vi "LoopselFFBlock.VI"() -> ()   [LabVIEW 2015]
panel:
  in  "no.of blocks":u32=2
  out "SEC":dbl=0.0202
  out "MB RAM":u32=4
  in  "?":enum32{"1", "2", "3"}(radio)=enum."3"
  in  "pos slope":u8=1
  in  "both slopes":u8
  in  "DAT in 10ns":u32
  out "FIFO overflow":bool
  in  "extTrig 0/1":u8
  in  "Start Read":bool
  in  "stop all":bool
  in  "Arm/Clear arry":bool
  in  "Slide":u32(slide)=1010 scale=996.0..1030.0
  in  "frequency[Hz]":u32
  in  "no.of samples (nos)":u32=1010
  in  "exposuretime[ms]":dbl=0.02 format="%.3f"
  out "Signalverlaufgraph":u16[](graph)=[542, 542, 543, 543, 0, 0, 1009, 0, 2, 2, 3, 3, 4, 4, 5, 5, 6, 6, 7, 7, 8, 8, 9, 9, 10, 10, 11, 11, 12, 12, 13, 13, 14, 14, 15, 15, 16, 16, 17, 17, 18, 18, 19, 19, 20, 20, 21, 21, 22, 22, 23, 23, 24, 24, 25, 25, 26, 26, 27, 27, 28, 28, 29, 29, 30, 30, 31, 31, 32, 32, 33, 33, 34, 34, 35, 35, 36, 36, 37, 37, 38, 38, 39, 39, 40, 40, 41, 41, 42, 42, 43, 43, 44, 44, 45, 45, 46, 46, 47, 47, 48, 48, 49, 49, 50, 50, 51, 51, 52, 52, 53, 53, 54, 54, 55, 55, 56, 56, 57, 57, 58, 58, 59, 59, 60, 60, 61, 61, 62, 62, 63, 63, 64, 64, 65, 65, 66, 66, 67, 67, 68, 68, 69, 69, 70, 70, 71, 71, 72, 72, 73, 73, 74, 74, 75, 75, 76, 76, 77, 77, 78, 78, 79, 79, 80, 80, 81, 81, 82, 82, 83, 83, 84, 84, 85, 85, 86, 86, 87, 87, 88, 88, 89, 89, 90, 90, 91, 91, 92, 92, 93, 93, 94, 94, 95, 95, 96, 96, 97, 97, 98, 98, 99, 99, 100, 100, 101, 101, 102, 102, 103, 103, 104, 104, 105, 105, 106, 106, 107, 107, 108, 108, 109, 109, 110, 110, 111, 111, 112, 112, 113, 113, 114, 114, 115, 115, 116, 116, 117, 117, 118, 118, 119, 119, 120, 120, 121, 121, 122, 122, 123, 123, 124, 124, 125, 125, 126, 126, 127, 127, 128, 128, 129, 129, 130, 130, 131, 131, 132, 132, 133, 133, 134, 134, 135, 135, 136, 136, 137, 137, 138, 138, 139, 139, 140, 140, 141, 141, 142, 142, 143, 143, 144, 144, 145, 145, 146, 146, 147, 147, 148, 148, 149, 149, 150, 150, 151, 151, 152, 152, 153, 153, 154, 154, 155, 155, 156, 156, 157, 157, 158, 158, 159, 159, 160, 160, 161, 161, 162, 162, 163, 163, 164, 164, 165, 165, 166, 166, 167, 167, 168, 168, 169, 169, 170, 170, 171, 171, 172, 172, 173, 173, 174, 174, 175, 175, 176, 176, 177, 177, 178, 178, 179, 179, 180, 180, 181, 181, 182, 182, 183, 183, 184, 184, 185, 185, 186, 186, 187, 187, 188, 188, 189, 189, 190, 190, 191, 191, 192, 192, 193, 193, 194, 194, 195, 195, 196, 196, 197, 197, 198, 198, 199, 199, 200, 200, 201, 201, 202, 202, 203, 203, 204, 204, 205, 205, 206, 206, 207, 207, 208, 208, 209, 209, 210, 210, 211, 211, 212, 212, 213, 213, 214, 214, 215, 215, 216, 216, 217, 217, 218, 218, 219, 219, 220, 220, 221, 221, 222, 222, 223, 223, 224, 224, 225, 225, 226, 226, 227, 227, 228, 228, 229, 229, 230, 230, 231, 231, 232, 232, 233, 233, 234, 234, 235, 235, 236, 236, 237, 237, 238, 238, 239, 239, 240, 240, 241, 241, 242, 242, 243, 243, 244, 244, 245, 245, 246, 246, 247, 247, 248, 248, 249, 249, 250, 250, 251, 251, 252, 252, 253, 253, 254, 254, 255, 255, 256, 256, 257, 257, 258, 258, 259, 259, 260, 260, 261, 261, 262, 262, 263, 263, 264, 264, 265, 265, 266, 266, 267, 267, 268, 268, 269, 269, 270, 270, 271, 271, 272, 272, 273, 273, 274, 274, 275, 275, 276, 276, 277, 277, 278, 278, 279, 279, 280, 280, 281, 281, 282, 282, 283, 283, 284, 284, 285, 285, 286, 286, 287, 287, 288, 288, 289, 289, 290, 290, 291, 291, 292, 292, 293, 293, 294, 294, 295, 295, 296, 296, 297, 297, 298, 298, 299, 299, 300, 300, 301, 301, 302, 302, 303, 303, 304, 304, 305, 305, 306, 306, 307, 307, 308, 308, 309, 309, 310, 310, 311, 311, 312, 312, 313, 313, 314, 314, 315, 315, 316, 316, 317, 317, 318, 318, 319, 319, 320, 320, 321, 321, 322, 322, 323, 323, 324, 324, 325, 325, 326, 326, 327, 327, 328, 328, 329, 329, 330, 330, 331, 331, 332, 332, 333, 333, 334, 334, 335, 335, 336, 336, 337, 337, 338, 338, 339, 339, 340, 340, 341, 341, 342, 342, 343, 343, 344, 344, 345, 345, 346, 346, 347, 347, 348, 348, 349, 349, 350, 350, 351, 351, 352, 352, 353, 353, 354, 354, 355, 355, 356, 356, 357, 357, 358, 358, 359, 359, 360, 360, 361, 361, 362, 362, 363, 363, 364, 364, 365, 365, 366, 366, 367, 367, 368, 368, 369, 369, 370, 370, 371, 371, 372, 372, 373, 373, 374, 374, 375, 375, 376, 376, 377, 377, 378, 378, 379, 379, 380, 380, 381, 381, 382, 382, 383, 383, 384, 384, 385, 385, 386, 386, 387, 387, 388, 388, 389, 389, 390, 390, 391, 391, 392, 392, 393, 393, 394, 394, 395, 395, 396, 396, 397, 397, 398, 398, 399, 399, 400, 400, 401, 401, 402, 402, 403, 403, 404, 404, 405, 405, 406, 406, 407, 407, 408, 408, 409, 409, 410, 410, 411, 411, 412, 412, 413, 413, 414, 414, 415, 415, 416, 416, 417, 417, 418, 418, 419, 419, 420, 420, 421, 421, 422, 422, 423, 423, 424, 424, 425, 425, 426, 426, 427, 427, 428, 428, 429, 429, 430, 430, 431, 431, 432, 432, 433, 433, 434, 434, 435, 435, 436, 436, 437, 437, 438, 438, 439, 439, 440, 440, 441, 441, 442, 442, 443, 443, 444, 444, 445, 445, 446, 446, 447, 447, 448, 448, 449, 449, 450, 450, 451, 451, 452, 452, 453, 453, 454, 454, 455, 455, 456, 456, 457, 457, 458, 458, 459, 459, 460, 460, 461, 461, 462, 462, 463, 463, 464, 464, 465, 465, 466, 466, 467, 467, 468, 468, 469, 469, 470, 470, 471, 471, 472, 472, 473, 473, 474, 474, 475, 475, 476, 476, 477, 477, 478, 478, 479, 479, 480, 480, 481, 481, 482, 482, 483, 483, 484, 484, 485, 485, 486, 486, 487, 487, 488, 488, 489, 489, 490, 490, 491, 491, 492, 492, 493, 493, 494, 494, 495, 495, 496, 496, 497, 497, 498, 498, 499, 499, 500, 500, 501, 501, 502, 502, 503, 503, 504, 504, 505, 505, 506, 506, 507, 507, 508, 508, 509, 509, 510, 510, 511, 511, 512, 512, 513, 513, 514, 514, 515, 515, 516, 516, 517, 517, 518, 518, 519, 519, 520, 520, 521, 521, 522, 522, 523, 523, 524, 524, 525, 525, 526, 526, 527, 527, 528, 528, 529, 529, 530, 530, 531, 531, 532, 532, 533, 533, 534, 534, 535, 535, 536, 536, 537, 537, 538, 538, 539, 539, 540, 540, 541, 541]
  # "Start with run"
  # "Abort with ESC"
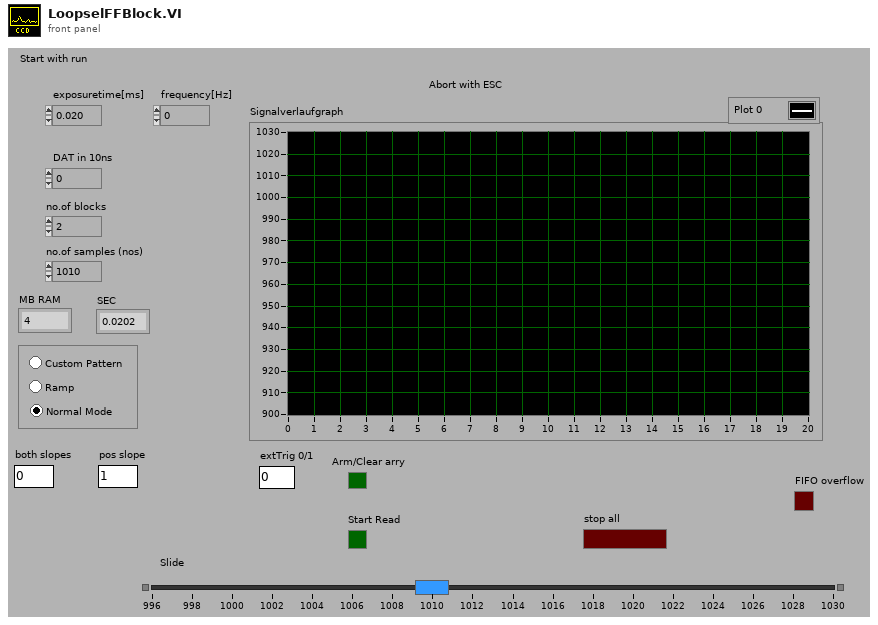
[diagram p1: front panel]
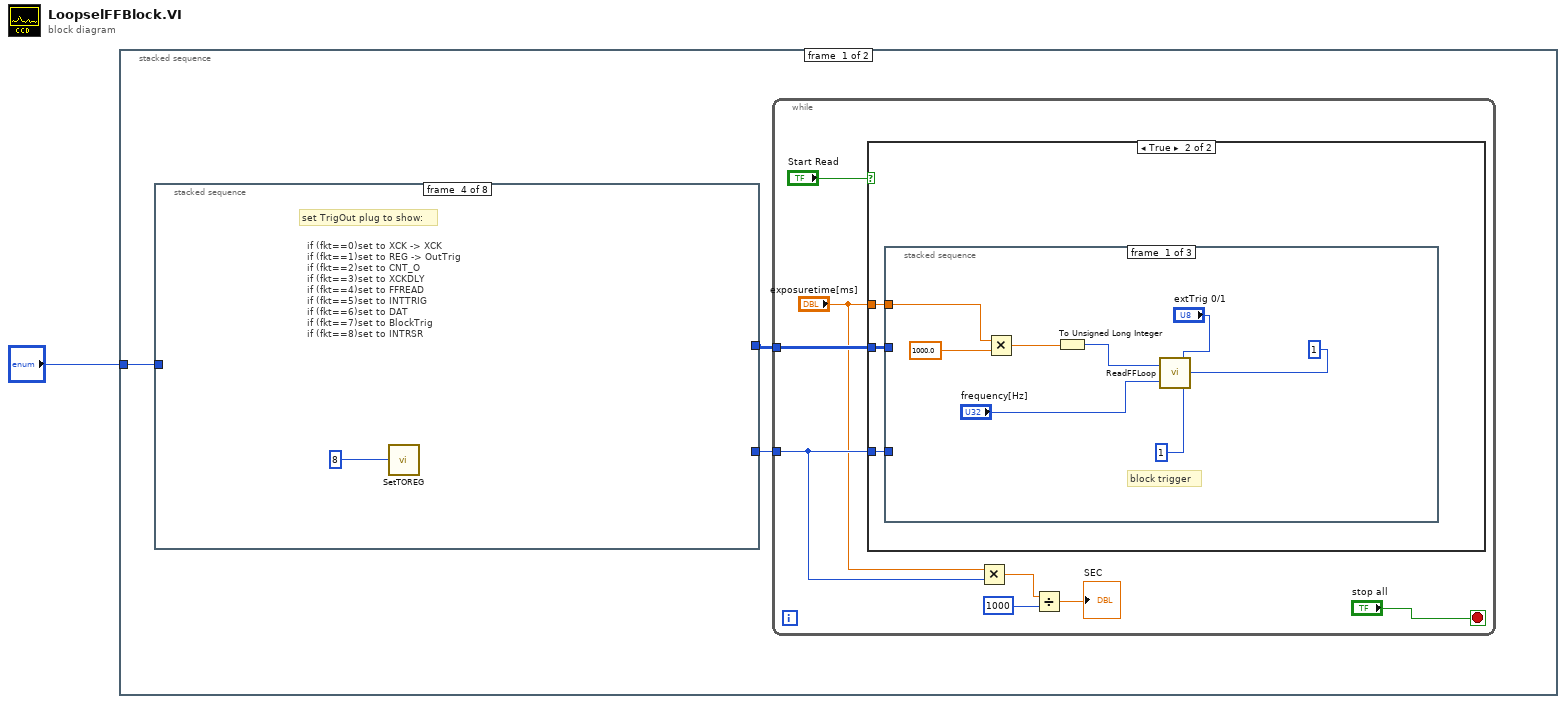
[diagram p0: block diagram]
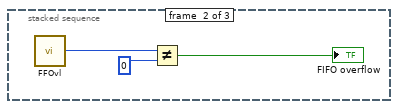
[diagram p3: hidden frame]
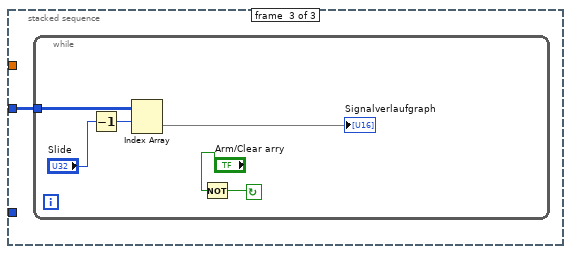
[diagram p4: hidden frame]
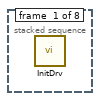
[diagram p5: hidden frame]
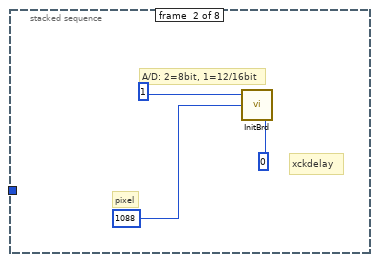
[diagram p6: hidden frame]
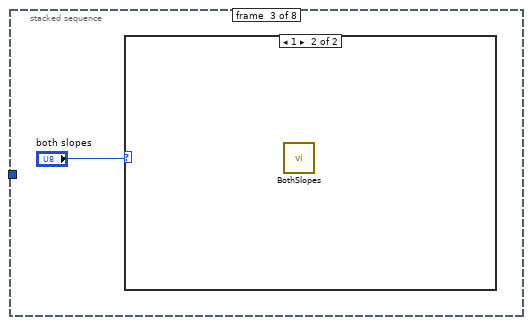
[diagram p7: hidden frame]
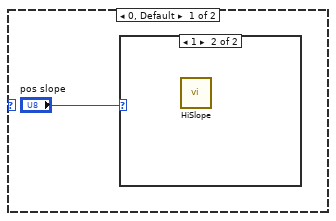
[diagram p8: hidden frame]
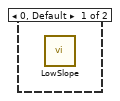
[diagram p9: hidden frame]
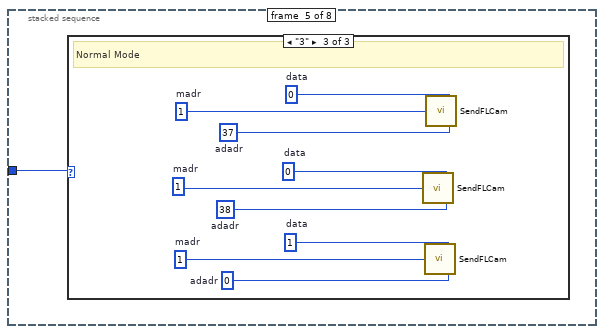
[diagram p10: hidden frame]
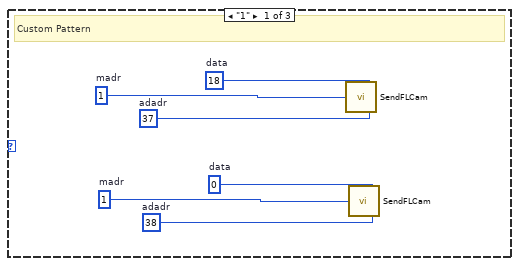
[diagram p11: hidden frame]
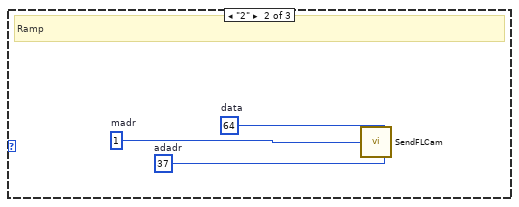
[diagram p12: hidden frame]
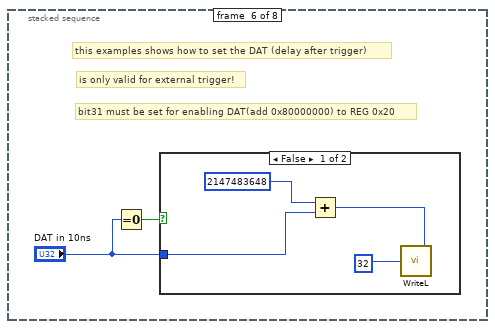
[diagram p13: hidden frame]
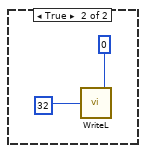
[diagram p14: hidden frame]
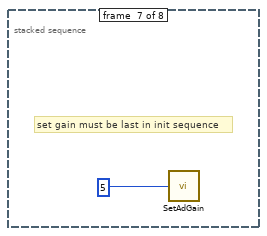
[diagram p15: hidden frame]
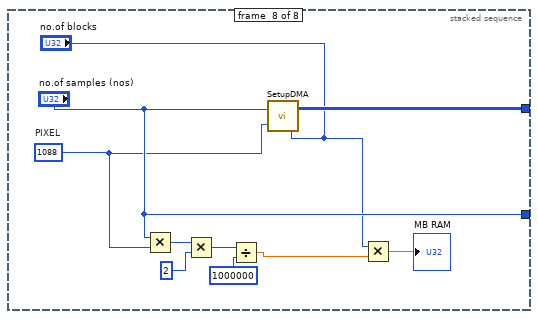
[diagram p16: hidden frame]
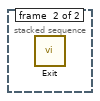
[diagram p17: hidden frame]
diagram:
  n1 = stacked-sequence {
    tunnel: "?" -> [w3 _]
    frame #0 {
      n2 = stacked-sequence {
        tunnel: [_ _ _ _ _ _ _ w73] -> w4
        tunnel: w3 -> [_ _ _ _ w40 _ _ _]
        tunnel: [_ _ _ _ _ _ _ "no.of samples (nos)"] -> w2
        frame #0 {
          n3 = call "InitDrv.vi"() -> ()  [unwired: 1 in]
        }
        frame #1 {
          # "pixel"
          # "xckdelay"
          # "A/D: 2=8bit, 1=12/16bit"
          n4 = call "InitBrd.vi"("xckdly"=u32 0, "pixel"=u32 1088, "flag816"=u32 1) -> ()  [unwired: 3 in]
        }
        frame #2 {
          n5 = case shown="1" "both slopes" {
            frame 0, Default {
              n6 = case shown="1" "pos slope" {
                frame 0, Default {
                  n7 = call "LowSlope.vi"() -> ()  [unwired: 1 in]
                }
                frame 1 {
                  n8 = call "HiSlope.vi"() -> ()  [unwired: 1 in]
                }
              }
            }
            frame 1 {
              n9 = call "BothSlopes.vi"() -> ()  [unwired: 1 in]
            }
          }
        }
        frame #3 {
          # "set TrigOut plug to show:"
          # "if (fkt==0)set to XCK -> XCK\nif (fkt==1)set to REG -> OutTrig\nif (fkt==2)set to CNT_O\nif (fkt==3)set to XCKDLY\nif (fkt==4)set to FFREAD\nif (fkt==5)set to INTTRIG\nif (fkt==6)set to DAT\nif (fkt==7)set to BlockTrig\nif (fkt==8)set to INTRSR"
          n10 = call "SetTOREG.vi"("fkt"=u8 8) -> ()
        }
        frame #4 {
          n11 = case shown="\"3\"" w40 {
            frame "1" {
              w41 = 0  # data
              w42 = 38  # adadr
              w43 = 1  # madr
              w44 = 18  # data
              w45 = 37  # adadr
              w46 = 1  # madr
              # "Custom Pattern"
              n12 = call "SendFLCam.vi"("madr"=w46, "data"=w44, "adadr"=w45) -> ()
              n13 = call "SendFLCam.vi"("madr"=w43, "data"=w41, "adadr"=w42) -> ()
            }
            frame "2" {
              w47 = 64  # data
              w48 = 37  # adadr
              w49 = 1  # madr
              # "Ramp"
              n14 = call "SendFLCam.vi"("madr"=w49, "data"=w47, "adadr"=w48) -> ()
            }
            frame "3" {
              w50 = 1  # data
              w52 = 0  # adadr
              w51 = 1  # madr
              w55 = 0  # data
              w54 = 38  # adadr
              w53 = 1  # madr
              w58 = 0  # data
              w57 = 37  # adadr
              w56 = 1  # madr
              # "Normal Mode"
              n15 = call "SendFLCam.vi"("madr"=w53, "data"=w55, "adadr"=w54) -> ()
              n16 = call "SendFLCam.vi"("madr"=w51, "data"=w50, "adadr"=w52) -> ()
              n17 = call "SendFLCam.vi"("madr"=w56, "data"=w58, "adadr"=w57) -> ()
            }
          }
        }
        frame #5 {
          # "bit31 must be set for enabling DAT(add 0x80000000) to REG 0x20"
          # "is only valid for external trigger!"
          # "this examples shows how to set the DAT (delay after trigger)"
          n18 = Equal To 0?(x="DAT in 10ns") -> (x = 0?=w60:bool)
          n19 = case shown="False" w60 {
            tunnel: "DAT in 10ns" -> [w61 _]
            frame False {
              n20 = Add(x=u32 2147483648, y=w61) -> (x+y=w64:u32)
              n21 = call "WriteL.vi"("val"=w64, "offset"=u32 32) -> ()
            }
            frame True {
              n22 = call "WriteL.vi"("val"=0, "offset"=u32 32) -> ()
            }
          }
        }
        frame #6 {
          # "set gain must be last in init sequence"
          n23 = call "SetAdGain.vi"("gain"=u8 5) -> ()  [unwired: 1 in]
        }
        frame #7 {
          w71 = u32 1088  # PIXEL
          n24 = Multiply(x="no.of samples (nos)", y=w71) -> (x*y=w77:u32)
          n25 = Multiply(x=w77, y=2) -> (x*y=w76:u32)
          n26 = Divide(x=w76, y=1000000) -> (x/y=w68:dbl)
          n27 = call "SetupDMA.vi"("blocks"="no.of blocks", "pixel"=w71, "nos"="no.of samples (nos)") -> ("Data Values"=w73:u16[][])
          n28 = Multiply(x="no.of blocks", y=w68) -> (x*y=→"MB RAM":dbl)
        }
      }
      n29 = while {
        tunnel: w4 -> [w12]
        tunnel: w2 -> [w7]
        stop <- "stop all" stop-if-true
        n30 = case shown="True" "Start Read" {
          tunnel: w12 -> [_ w15]
          tunnel: w7 -> [_ w14]
          tunnel: "exposuretime[ms]" -> [_ w13]
          frame False {
          }
          frame True {
            n31 = stacked-sequence {
              tunnel: w15 -> [_ _ w27]
              tunnel: w14 -> [_ _ _]
              tunnel: w13 -> [w16 _ _]
              frame #0 {
                # "block trigger"
                n32 = Multiply(x=w16, y=1000.0) -> (x*y=w17:dbl)
                n33 = To Unsigned Long Integer(number=w17) -> (unsigned 32bit integer=w22:u32)
                n34 = call "ReadFFLoop.vi"("exptus"=w22, "freq"="frequency[Hz]", "ExtTrig"="extTrig 0/1", "btrig_ch"=u8 1, "blocktrigger"=u8 1) -> ()
              }
              frame #1 {
                n35 = call "FFOvl.vi"() -> ("FFOvl"=w25:u8)  [unwired: 1 in]
                n36 = Not Equal?(x=w25, y=0) -> (x != y?=→"FIFO overflow":bool)
              }
              frame #2 {
                n37 = while {
                  tunnel: w27 -> [w30]
                  stop <- w33 continue-if-true
                  n38 = Decrement(x="Slide") -> (x-1=w32:u32)
                  n39 = Index Array(array=w30, index (row)=w32) -> (element=→"Signalverlaufgraph":u16[])  [unwired: 1 in]
                  n40 = Not(x="Arm/Clear arry") -> (.not. x?=w33:bool)
                }
              }
            }
          }
        }
        n41 = Multiply(x="exposuretime[ms]", y=w7) -> (x*y=w9:dbl)
        n42 = Divide(x=w9, y=1000) -> (x/y=→"SEC":dbl)
      }
    }
    frame #1 {
      n43 = call "Exit.vi"() -> ()  [unwired: 1 in]
    }
  }
